vi "Get Value (Boolean[]).vi"(8 "error in (no error)":errorcluster, 10 "Keys":string[](array[string]), 11 "JSON Value in":refnum<class "JSON Value.lvclass">) -> (0 "error out":errorcluster, 2 "value":bool)   [LabVIEW 2016, in "JSON Value.lvclass"]
uses:
  JSON Value.lvclass
  Get Value (Value[]).vi
  Read Value/Read value (Boolean).vi
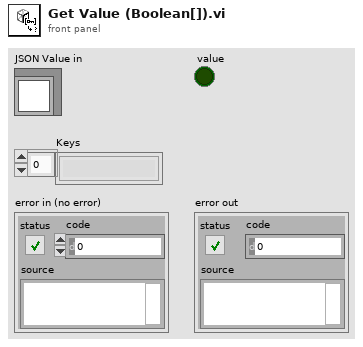
[diagram p1: front panel]
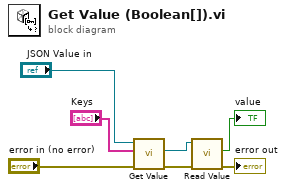
[diagram p0: block diagram]
diagram:
  n1 = call-poly "Get Value.vi"("error in (no error)"="error in (no error)", "Keys"="Keys", "JSON Value in"="JSON Value in") -> ("error out"=w5:errorcluster, "JSON Value out"=w4:refnum<class "JSON Value.lvclass">)  [unwired: 7 in]
  n2 = call-poly "Read Value.vi"("error in (no error)"=w5, "JSON Boolean in"=w4) -> ("error out"=→"error out":errorcluster, "value"=→"value":bool)  [unwired: 8 in]
